vi "updateZkAndDofIdx.vi"(8 "error in (no error)":errorcluster, 11 "OptStateEsti in":refnum<class "OptStateEsti.lvclass">) -> (0 "error out":errorcluster, 3 "OptStateEsti out":refnum<class "OptStateEsti.lvclass">)   [LabVIEW 2016, in "OptStateEsti.lvclass"]
uses:
  OptStateEsti.lvclass
panel:
  in  "Array":dbl[](array[numeric])
  in  "zn3Idx":bool[](array[boolean])
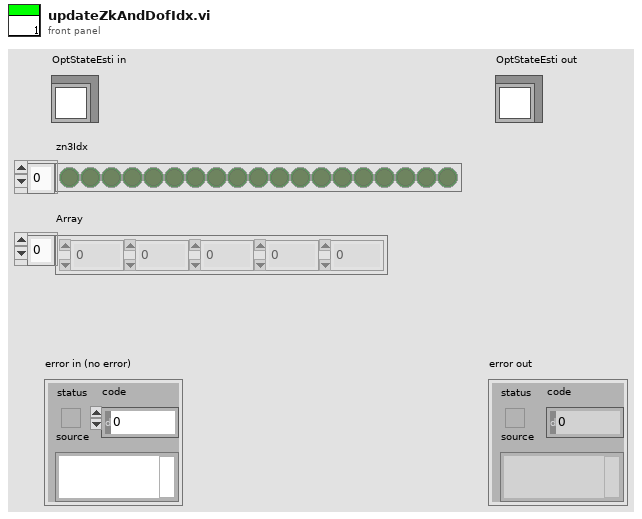
[diagram p1: front panel]
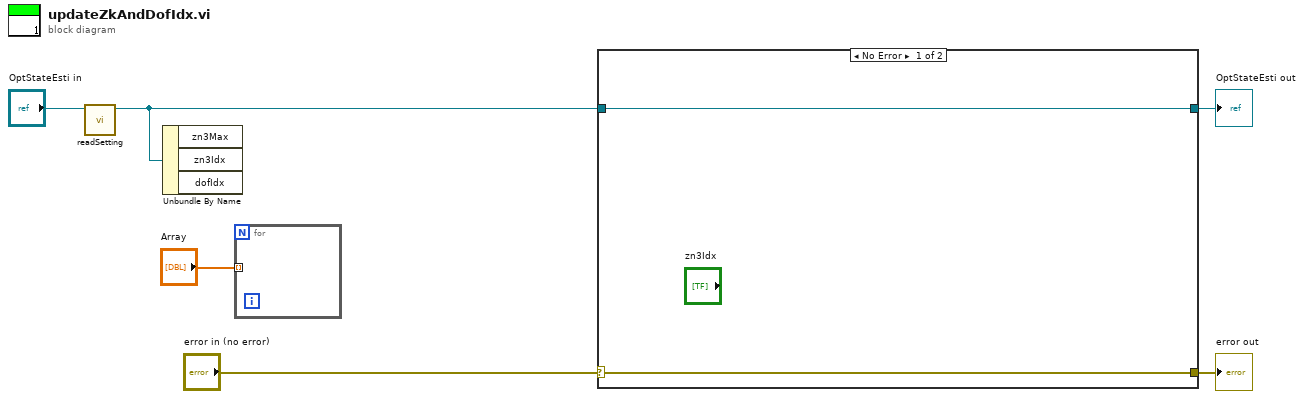
[diagram p0: block diagram]
diagram:
  n1 = call "readSetting.vi"("OptStateEsti in"="OptStateEsti in") -> ("OptStateEsti out"=w2:refnum<class "OptStateEsti.lvclass">)  [unwired: 9 in, 1 out]
  n2 = Unbundle By Name(w2) -> ()  [unwired: 3 out]
  n3 = for {
    tunnel: "Array" -> [_] mode=indexing
  }
  n4 = case shown="No Error" "error in (no error)" {
    selector: "error in (no error)" -> [w7 w10]
    tunnel: [w7 w10] -> w5
    tunnel: [w8 w9] -> w4
    tunnel: w2 -> [w8 w9]
    frame No Error {
    }
    frame Error {
    }
  }
  "error out" <- w5
  "OptStateEsti out" <- w4
